vi "ATF-Pump-DI_Scale_Config.vi"(8 "error in (no error)":errorcluster, 10 "DI config":T1(array[cluster]), 11 "Refnum in":refnum<k21>) -> (0 "error out":errorcluster, 3 "Refnum out":refnum<k21>)   [LabVIEW 2022 SP3]
uses:
  <vilib>/DAQmx/create/channels.llb/DAQmx Create Channel (DI-Digital Input).vi
  <resource>/objmgr/daqmx.rc
panel:
  out "Array":bool[](array[boolean])
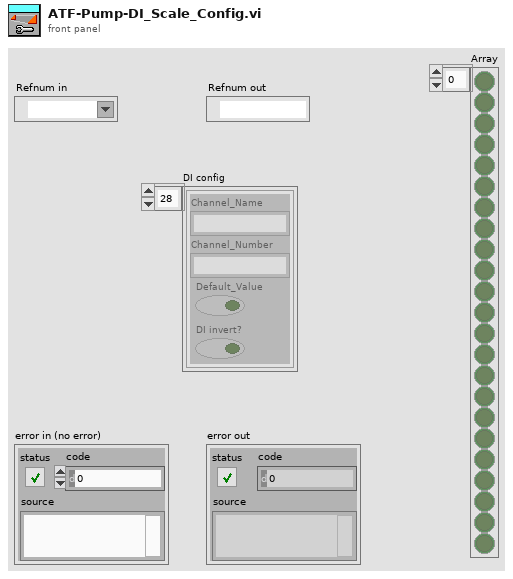
[diagram p1: front panel]
types:
  T1 = cluster{"Channel_Name":string, "Channel_Number":string, "Default_Value":bool, "DI invert?":bool}[]
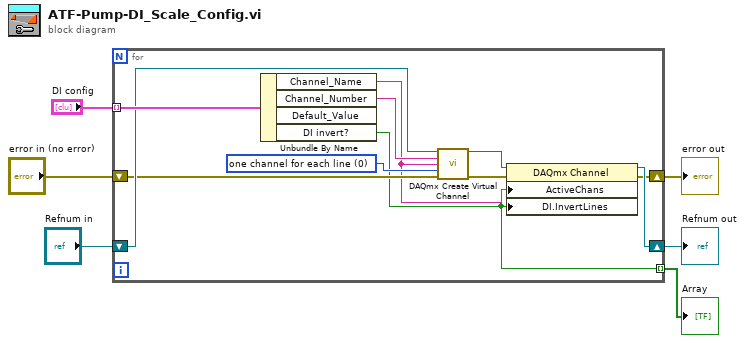
[diagram p0: block diagram]
diagram:
  n1 = for {
    tunnel: "DI config" -> [w17] mode=indexing
    shift-right: [w10] -> w3
    shift-left: "Refnum in" -> [w16]
    shift-right: [w9] -> w4
    shift-left: "error in (no error)" -> [w15]
    tunnel: [w7] -> w1 mode=indexing
    w13 = 0 items=["one channel for each line", "one channel for all lines"] ("line grouping")
    n2 = Unbundle By Name(w17) -> ("Channel_Name"=w8:string, "Channel_Number"=w14:string, "DI invert?"=w7:bool)  [unwired: 1 out]
    n3 = call-poly <vilib>:"DAQmx Create Virtual Channel.vi"("task in"=w16, "lines"=w14, "name to assign"=w8, "line grouping"=w13, "error in"=w15) -> ("task out"=w12:refnum<k21>, "error out"=w11:errorcluster)  [unwired: 9 in]
    n4 = property on="Property Node" class="DAQmx Channel"(reference=w12, error in=w11, "ActiveChans"=w8, "DI.InvertLines"=w7) -> (reference out=w10:refnum<k21>, error out=w9:errorcluster)
  }
  "error out" <- w4
  "Refnum out" <- w3
  "Array" <- w1
